vi "Export String to Clipboard.vi"(8 "error in":errorcluster, 11 "string":string) -> (0 "error out":errorcluster)   [LabVIEW 2010]
doc: "Export the string value to the Operating System Clipboard."
panel:
  out "string array":string[](array[string])
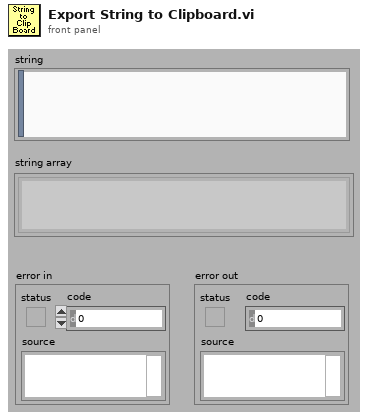
[diagram p1: front panel]
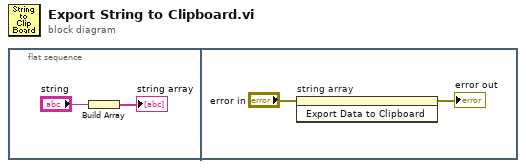
[diagram p0: block diagram]
diagram:
  n1 = flat-sequence {
    frame #0 {
      n2 = Build Array("string") -> (→"string array":string[])
    }
    frame #1 {
      n3 = invoke on="string array" class="Arr (strict)" method="Export Data to Clipboard"(error in="error in") -> (error out=→"error out":errorcluster)  [unwired: 2 in, 2 out]
    }
  }
